vi "MainForceMeasurement.vi"() -> ()   [LabVIEW 2010]
uses:
  <vilib>/Instr/_visa.llb/VISA Flush IO Buffer Mask.ctl
  Variable globale 1.vi
  <vilib>/Instr/_visa.llb/VISA Configure Serial Port (Instr).vi
panel:
  in  "attente (ms)":u32=50
  in  "Temps échelon":i32=25
  out "Sor":string[][](array[string]) caption="Motor torque"
  out "Ent":string[][](array[string]) caption="Motor commande"
  out "Con_XYLeftTorque 2":cluster{"Y":dbl[], "Y":dbl[]}[](graph) caption="Motor Torque"
  out "Con_XYLeftTorque":cluster{"Y":dbl[], "Y":dbl[]}[](graph) caption="Motor  Torque command"
  in  "Temps départ":i32=25
  out "tableau inversé 2":u8[](array[numeric])
  out "tableau inversé":i8[](array[numeric])
  out "error out 2":errorcluster caption="sortie d'erreur"
  in  "Type moteur":i32=139 min=0 max=255
  out "Float recu":sgl
  in  "Couple":sgl=25.45
  out "Iteration 3":i32
  out "Iteration reception":i32
  out "Iteration Envoi":i32
  out "Checksum calculé":i32
  out "Checksum reçu":i32
  out "Type de donnee (ID)":i32
  out "Byte Start ?":bool
  out "Retour 2":string
  in  "stop secu":bool
  in  "STOP":bool
  out "error out":errorcluster caption="sortie d'erreur"
  in  "baud rate (9600)":u32=9600 caption="débit en bauds (9600)"
  in  "Port Com":refnum<visa-resource-name>="COM7" caption="Nom de ressource VISA"
  # "Envoi de l'échelon"
  # "Réception"
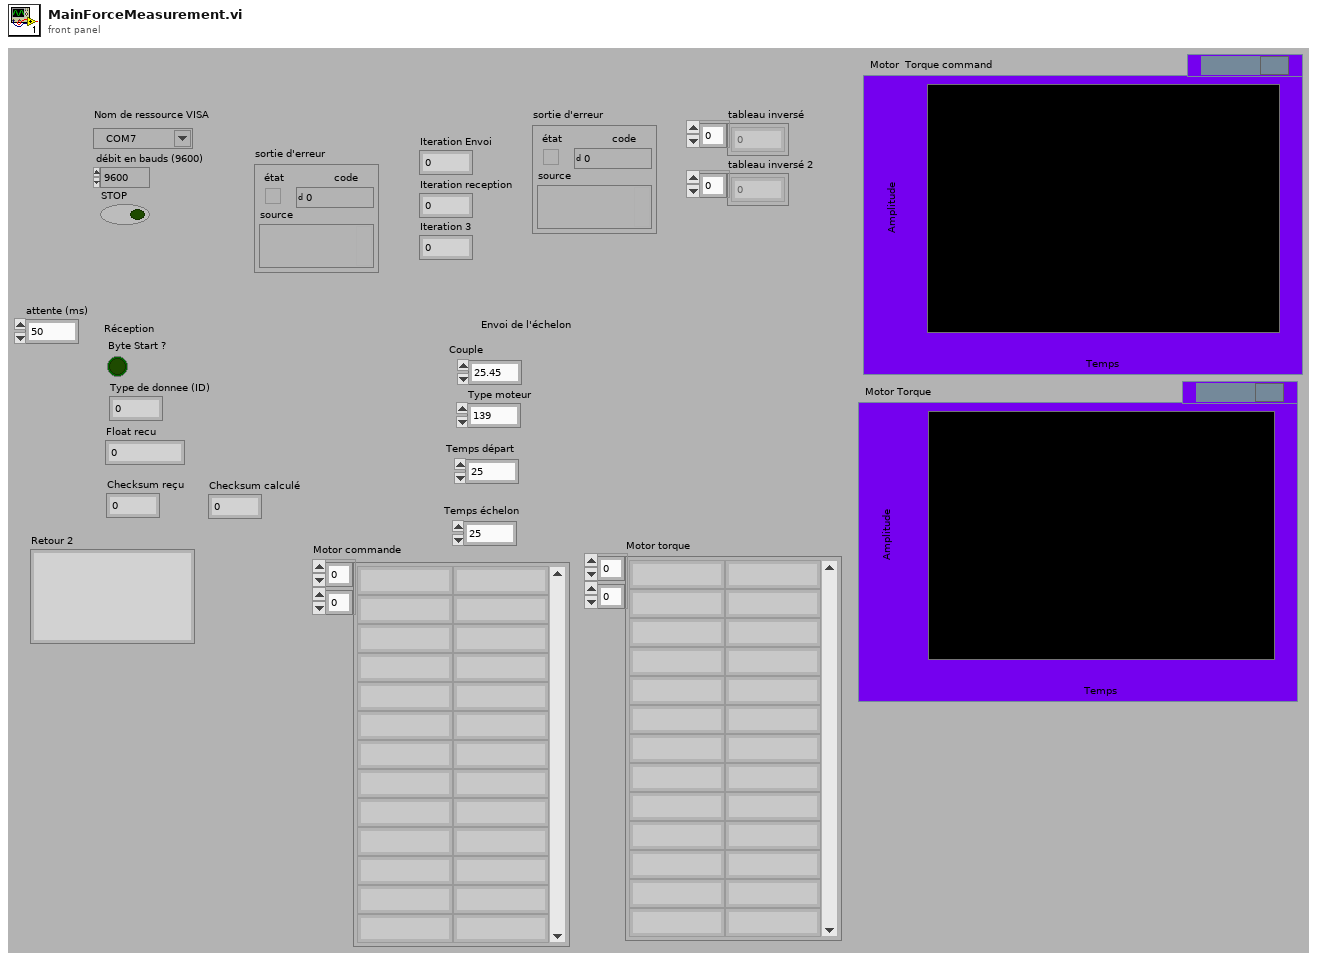
[diagram p1: front panel]
types:
  T1 = typedef "VISA Flush IO Buffer Mask.ctl" = u16
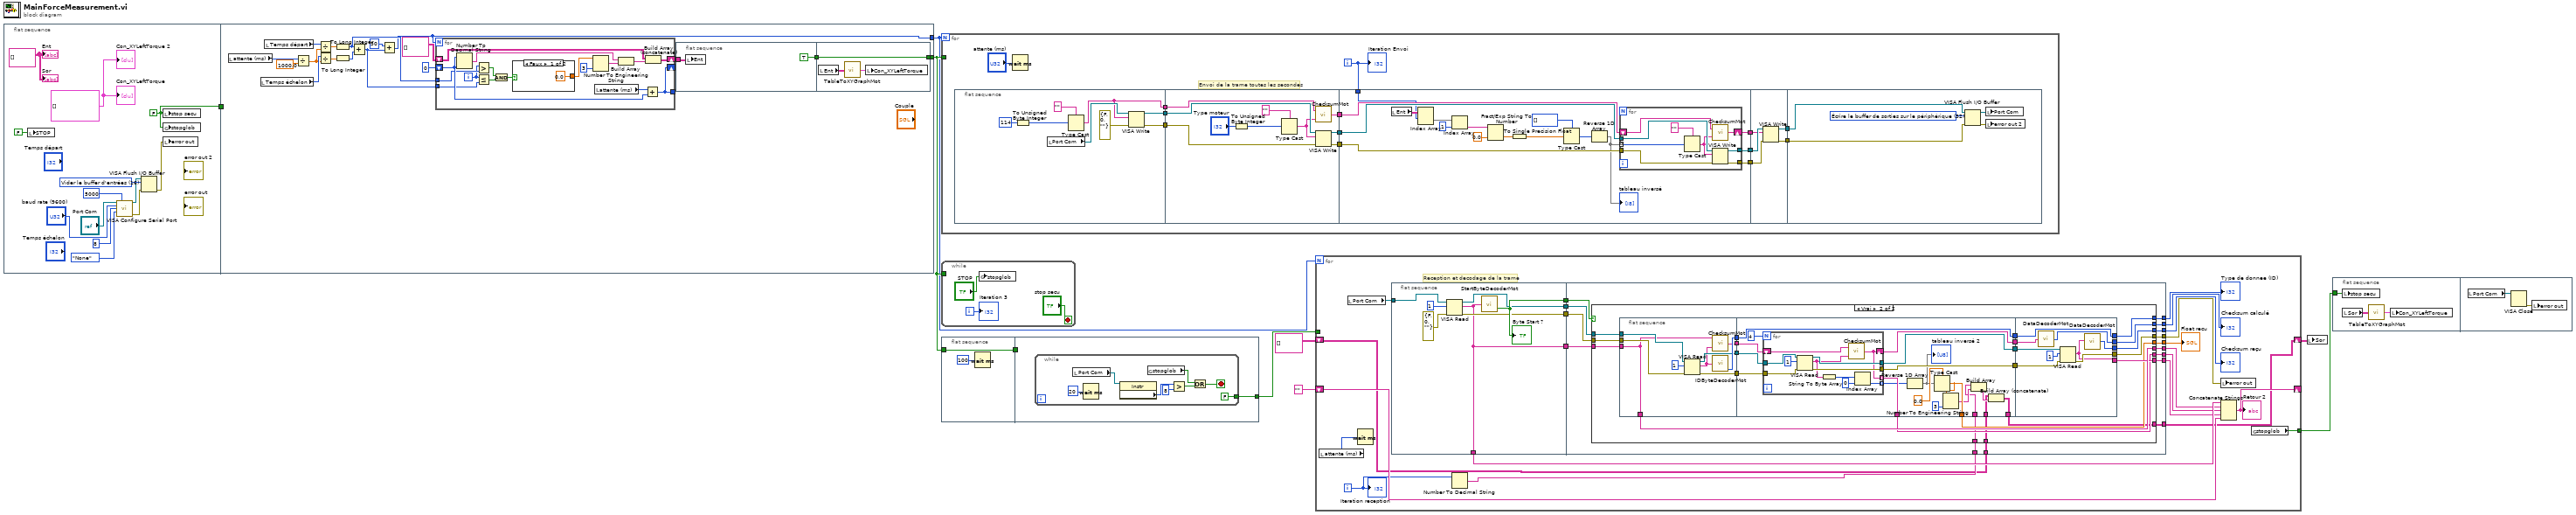
[diagram p0: block diagram]
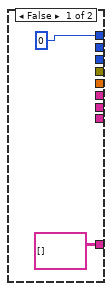
[diagram p2: hidden frame]
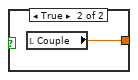
[diagram p3: hidden frame]
diagram:
  n1 = flat-sequence {
    tunnel: [w14] -> w5
    tunnel: [w31] -> w8
    tunnel: w5 -> [_]
    tunnel: [w26] -> w3
    frame #0 {
      w11 = cluster{"Y":dbl[], "Y":dbl[]}[] [] ("Con_XYLeftTorque 2")
      w10 = string[][] [] ("Con_MotorRightTorque")
      w14 = FALSE
      w17 = T1 16 items=["Vider le buffer d'entrées"=16, "Écrire le buffer de sorties sur le périphérique"=32, "Vider le buffer d'entrées (Pas d'E/S)"=64, "Vider le buffer de sorties"=128] ("Mask")
      n2 = local write "STOP"(FALSE) -> ()
      n3 = call-poly "VISA Configure Serial Port"("VISA resource name"="Port Com", "timeout (10sec)"=u32 5000, "baud rate (9600)"="baud rate (9600)", "data bits (8)"=u16 8, "parity (0:none)"=enum16{"None", "Odd", "Even", "Mark", "Space"}."None") -> ("VISA resource name out"=w13:refnum<visa-resource-name>, "error out"=w12:errorcluster)  [unwired: 9 in]
      n4 = VISA Flush I/O Buffer(VISA resource name=w13, mask (16)=w17, error in (no error)=w12) -> (error out=w15:errorcluster)  [unwired: 1 out]
      n5 = local write "stop secu"(w14) -> ()
      n6 = global write "Variable globale 1.vi" "stopglob"(w14) -> ()
      n7 = local write "error out"(w15) -> ()
      "Sor" <- w10
      "Con_XYLeftTorque" <- w11
      "Con_XYLeftTorque 2" <- w11
      "Ent" <- w10
    }
    frame #1 {
      n8 = local read "attente (ms)"() -> (w29:u32)
      n9 = local read "Temps échelon"() -> (w37:i32)
      n10 = local read "Temps départ"() -> (w39:i32)
      n11 = Divide(x=w29, y=sgl 1000.0) -> (x/y=w30:sgl)
      n12 = Divide(x=w39, y=w30) -> (x/y=w38:sgl)
      n13 = Divide(x=w37, y=w30) -> (x/y=w36:sgl)
      n14 = To Long Integer(number=w38) -> (32bit integer=w32:i32)
      n15 = To Long Integer(number=w36) -> (32bit integer=w35:i32)
      n16 = Add(x=w32, y=w35) -> (x+y=w24:i32)
      n17 = Add(x=50, y=w24) -> (x+y=w26:i32)
      n18 = for {
        N: w26 -> [_]
        shift-right: [w51] -> w27
        shift-left: string[][] [] ("Ent") -> [w52]
        shift-right: [w50] -> _
        shift-left: u32 0 -> [w60]
        tunnel: w32 -> [w58]
        tunnel: [w50] -> _
        tunnel: w24 -> [w48]
        i -> [w49]
        n19 = Number To Decimal String(number=w60) -> (decimal integer string=w57:string)  [unwired: 1 in]
        n20 = Greater?(x=w49, y=w58) -> (0:w47:bool)
        n21 = Less Or Equal?(x=w49, y=w48) -> (x <= y?=w46:bool)
        n22 = And(x=w47, y=w46) -> (x .and. y?=w45:bool)
        n23 = case shown="Faux" w45 {
          tunnel: [sgl 0.0 ("Couple") w62] -> w55
          frame False {
          }
          frame True {
            n24 = local read "Couple"() -> (w62:sgl)
          }
        }
        n25 = Number To Engineering String(2:i16 3 ("précision (6)"), 4:w55) -> (0:w56:string)  [unwired: 2 in]
        n26 = local read "attente (ms)"() -> (w59:u32)
        n27 = Build Array(w57, w56) -> (w53:string[])
        n28 = Add(x=w59, y=w60) -> (x+y=w50:u32)
        n29 = Build Array (concatenate)(w52, w53) -> (w51:string[][])
      }
      n30 = flat-sequence {
        tunnel: w27 -> [w40]
        tunnel: [TRUE] -> w23
        tunnel: [w44] -> w31
        tunnel: w23 -> [w44]
        frame #0 {
          n31 = local write "Ent"(w40) -> ()
        }
        frame #1 {
          n32 = local read "Ent"() -> (w42:string[][])
          n33 = call "TableToXYGraphMot.vi"("Input Table"=w42) -> ("XY Graph"=w43:cluster{"Y":dbl[], "Y":dbl[]}[])
          n34 = local write "Con_XYLeftTorque"(w43) -> ()
        }
      }
    }
  }
  n35 = for {
    N: w3 -> [_]
    tunnel: w8 -> [_]
    i -> [w63]
    # "Envoi de la trame toutes les secondes"
    n36 = flat-sequence {
      tunnel: [w80] -> w75
      tunnel: [w79] -> w74
      tunnel: [w78] -> w71
      tunnel: w75 -> [w93]
      tunnel: w74 -> [w92]
      tunnel: [w91] -> w73
      tunnel: [w90] -> w72
      tunnel: w71 -> [w89]
      tunnel: [w88] -> w70
      tunnel: w73 -> [w107]
      tunnel: w72 -> [w109]
      tunnel: w70 -> [w105]
      tunnel: [w108] -> w69
      tunnel: [w106] -> w68
      tunnel: [w104] -> w67
      tunnel: w63 -> [w100]
      tunnel: w69 -> [w124]
      tunnel: w68 -> [w123]
      tunnel: w67 -> [w122]
      tunnel: [w121] -> w65
      tunnel: [w120] -> w64
      tunnel: w65 -> [w129]
      tunnel: w64 -> [w128]
      frame #0 {
        n37 = To Unsigned Byte Integer(number=114) -> (unsigned 8bit integer=w77:u8)
        n38 = local read "Port Com"() -> (w83:refnum<visa-resource-name>)
        n39 = Type Cast(type="", x=w77) -> (*(type *) &x=w78:string)
        n40 = VISA Write(VISA resource name=w83, write buffer=w78, error in (no error)=errorcluster {"status"=FALSE, "code"=0, "source"=""} ("entrée d'erreur (pas d'erreur)")) -> (VISA resource name out=w80:refnum<visa-resource-name>, error out=w79:errorcluster)  [unwired: 1 out]
      }
      frame #1 {
        n41 = To Unsigned Byte Integer(number="Type moteur") -> (unsigned 8bit integer=w86:u8)
        n42 = Type Cast(type="", x=w86) -> (*(type *) &x=w84:string)
        n43 = call "ChecksumMot.vi"("Byte2"=w84, "Byte1"=w89) -> ("chaîne"=w88:string)
        n44 = VISA Write(VISA resource name=w93, write buffer=w84, error in (no error)=w92) -> (VISA resource name out=w90:refnum<visa-resource-name>, error out=w91:errorcluster)  [unwired: 1 out]
      }
      frame #2 {
        n45 = local read "Ent"() -> (w101:string[][])
        n46 = Index Array(array=w101, index (row)=w100) -> (element=w99:string[])  [unwired: 1 in]
        n47 = Index Array(array=w99, index=1 ("indice")) -> (element=w97:string)
        n48 = Fract/Exp String To Number(string=w97, default (0 dbl)=0.0 ("valeur par défaut (0 DBL)")) -> (number=w95:dbl)  [unwired: 2 in, 1 out]
        n49 = To Single Precision Float(number=w95) -> (single precision float=w94:sgl)
        n50 = Type Cast(type=i8[] [] ("tableau d'octets non signés"), x=w94) -> (*(type *) &x=w103:i8[])
        n51 = Reverse 1D Array(array=w103) -> (reversed array=w102:i8[])
        "tableau inversé" <- w102
        n52 = for {
          tunnel: w102 -> [w119] mode=indexing
          tunnel: w109 -> [w117]
          tunnel: [w116] -> w108
          tunnel: w107 -> [w115]
          tunnel: [w114] -> w106
          shift-right: [w111] -> w104
          shift-left: w105 -> [w113]
          n53 = Type Cast(type="", x=w119) -> (*(type *) &x=w112:string)
          n54 = call "ChecksumMot.vi"("Byte2"=w112, "Byte1"=w113) -> ("chaîne"=w111:string)
          n55 = VISA Write(VISA resource name=w117, write buffer=w112, error in (no error)=w115) -> (VISA resource name out=w116:refnum<visa-resource-name>, error out=w114:errorcluster)  [unwired: 1 out]
        }
      }
      frame #3 {
        n56 = VISA Write(VISA resource name=w124, write buffer=w122, error in (no error)=w123) -> (VISA resource name out=w121:refnum<visa-resource-name>, error out=w120:errorcluster)  [unwired: 1 out]
      }
      frame #4 {
        w125 = T1 32 items=["Vider le buffer d'entrées"=16, "Écrire le buffer de sorties sur le périphérique"=32, "Vider le buffer d'entrées (Pas d'E/S)"=64, "Vider le buffer de sorties"=128] ("Mask")
        n57 = VISA Flush I/O Buffer(VISA resource name=w129, mask (16)=w125, error in (no error)=w128) -> (VISA resource name out=w126:refnum<visa-resource-name>, error out=w127:errorcluster)
        n58 = local write "Port Com"(w126) -> ()
        n59 = local write "error out 2"(w127) -> ()
      }
    }
    n60 = Wait (ms)(milliseconds to wait="attente (ms)") -> ()  [unwired: 1 out]
    "Iteration Envoi" <- w63
  }
  n61 = while {
    tunnel: w8 -> [_]
    i -> [w130]
    stop <- "stop secu" stop-if-true
    n62 = global write "Variable globale 1.vi" "stopglob"("STOP") -> ()
    "Iteration 3" <- w130
  }
  n63 = flat-sequence {
    tunnel: w8 -> [w133]
    tunnel: [w133] -> w7
    tunnel: w7 -> [_]
    tunnel: [w135] -> w6
    frame #0 {
      n64 = Wait (ms)(milliseconds to wait=u32 100 ("attente (ms)")) -> ()  [unwired: 1 out]
    }
    frame #1 {
      n65 = while {
        tunnel: [FALSE] -> w135
        stop <- w142 stop-if-true
        n66 = local read "Port Com"() -> (w141:refnum<visa-resource-name>)
        n67 = Wait (ms)(milliseconds to wait=u32 20 ("attente (ms)")) -> ()  [unwired: 1 out]
        n68 = property class="Instr"(reference=w141) -> ("Serial Settings:Number of Bytes at Serial Port"=w140:u32)  [unwired: 1 in, 2 out]
        n69 = global read "Variable globale 1.vi" "stopglob"() -> (w143:bool)
        n70 = Greater?(x=w140, y=u32 8) -> (0:w138:bool)
        n71 = Or(x=w143, y=w138) -> (x .or. y?=w142:bool)
      }
    }
  }
  n72 = for {
    N: w3 -> [_]
    shift-right: [w151] -> _
    shift-left: "" -> [w152]
    tunnel: w6 -> [_]
    tunnel: [w148] -> w4
    shift-right: [w144] -> w1
    shift-left: string[][] [] ("Sor") -> [w145]
    i -> [w147]
    # "Reception et decodage de la trame"
    n73 = local read "attente (ms)"() -> (w165:u32)
    n74 = local read "Port Com"() -> (w164:refnum<visa-resource-name>)
    n75 = Wait (ms)(milliseconds to wait=w165) -> ()  [unwired: 1 out]
    n76 = flat-sequence {
      tunnel: w164 -> [w171]
      tunnel: [w170] -> w163
      tunnel: [w169] -> w162
      tunnel: [w168] -> w161
      tunnel: [w167] -> w159
      tunnel: [w167] -> w155
      tunnel: w163 -> [w187]
      tunnel: w162 -> [w186]
      tunnel: w161 -> [w185]
      tunnel: [w184] -> w160
      tunnel: w159 -> [w183]
      tunnel: [w182] -> w158
      tunnel: [w181] -> w157
      tunnel: [w180] -> w156
      tunnel: [w179] -> w154
      tunnel: [w178] -> w153
      tunnel: [w177] -> w150
      tunnel: [w176] -> w149
      tunnel: w146 -> [w175]
      tunnel: w145 -> [w174]
      tunnel: [w173] -> w144
      frame #0 {
        n77 = VISA Read(VISA resource name=w171, byte count=u32 1 ("nombre d'octets"), error in (no error)=errorcluster {"status"=FALSE, "code"=0, "source"=""} ("entrée d'erreur (pas d'erreur)")) -> (VISA resource name out=w169:refnum<visa-resource-name>, read buffer=w167:string, error out=w168:errorcluster)  [unwired: 1 out]
        n78 = call "StartByteDecoderMot.vi"("byte1"=w167) -> ("Byte Start ?"=w170:bool)  [unwired: 1 in]
        "Byte Start ?" <- w170
      }
      frame #1 {
        n79 = case shown="Vrai" w187 {
          tunnel: w186 -> [_ w211]
          tunnel: w185 -> [_ w210]
          tunnel: [0 ("Type de donnee (ID)") w209] -> w184
          tunnel: w183 -> [_ w204]
          tunnel: [_ w202] -> w182
          tunnel: [_ w201] -> w181
          tunnel: [_ w200] -> w180
          tunnel: [_ w199] -> w179
          tunnel: [_ w198] -> w178
          tunnel: [_ w195] -> w177
          tunnel: [_ w193] -> w176
          tunnel: w175 -> [_ w192]
          tunnel: w174 -> [_ w191]
          tunnel: [string[][] [] w190] -> w173
          frame False {
          }
          frame True {
            n80 = flat-sequence {
              tunnel: w211 -> [w220]
              tunnel: w210 -> [w219]
              tunnel: [w217] -> w208
              tunnel: [w216] -> w207
              tunnel: [w215] -> w206
              tunnel: w204 -> [w212]
              tunnel: [w213] -> w203
              tunnel: [w212] -> w199
              tunnel: w208 -> [w239]
              tunnel: w207 -> [w238]
              tunnel: w206 -> [w235]
              tunnel: [w239] -> w205
              tunnel: w203 -> [w233]
              tunnel: [w237] -> w197
              tunnel: [w236] -> w196
              tunnel: [w227] -> w195
              tunnel: [w232] -> w194
              tunnel: [w230] -> w193
              tunnel: w192 -> [w224]
              tunnel: w191 -> [w222]
              tunnel: [w221] -> w190
              tunnel: [w259] -> w209
              tunnel: w205 -> [w259]
              tunnel: [w257] -> w202
              tunnel: [w256] -> w201
              tunnel: [w255] -> w200
              tunnel: [w254] -> w198
              tunnel: w197 -> [w253]
              tunnel: w196 -> [w252]
              tunnel: w194 -> [w251]
              frame #0 {
                n81 = VISA Read(VISA resource name=w220, byte count=u32 1 ("nombre d'octets"), error in (no error)=w219) -> (VISA resource name out=w216:refnum<visa-resource-name>, read buffer=w214:string, error out=w215:errorcluster)  [unwired: 1 out]
                n82 = call "ChecksumMot.vi"("Byte2"=w214, "Byte1"=w212) -> ("chaîne"=w213:string)
                n83 = call "IDByteDecoderMot.vi"("byte1"=w214) -> ("Type de donnee (ID)"=w217:i32)  [unwired: 2 out]
              }
              frame #1 {
                n84 = for {
                  N: 4 -> [_]
                  tunnel: w238 -> [w249]
                  tunnel: [w248] -> w237
                  tunnel: [w247] -> w236
                  tunnel: w235 -> [w246]
                  tunnel: [w243] -> w229 mode=indexing
                  shift-right: [w240] -> w232
                  shift-left: w233 -> [w242]
                  tunnel: [w240] -> w230 mode=indexing
                  n85 = VISA Read(VISA resource name=w249, byte count=u32 1 ("nombre d'octets"), error in (no error)=w246) -> (VISA resource name out=w248:refnum<visa-resource-name>, read buffer=w241:string, error out=w247:errorcluster)  [unwired: 1 out]
                  n86 = String To Byte Array(string=w241) -> (unsigned byte array=w245:u8[])
                  n87 = call "ChecksumMot.vi"("Byte2"=w241, "Byte1"=w242) -> ("chaîne"=w240:string)
                  n88 = Index Array(array=w245, index=0 ("indice")) -> (element=w243:u8)
                }
                n89 = Reverse 1D Array(array=w229) -> (reversed array=w228:u8[])
                "tableau inversé 2" <- w228
                n90 = Type Cast(type=sgl 0.0, x=w228) -> (*(type *) &x=w227:sgl)
                n91 = Number To Engineering String(2:i16 3 ("précision (6)"), 4:w227) -> (0:w225:string)  [unwired: 2 in]
                n92 = Build Array(w224, w225) -> (w223:string[])
                n93 = Build Array (concatenate)(w222, w223) -> (w221:string[][])
              }
              frame #2 {
                n94 = call "DataDecoderMot.vi"("byte1"=w251) -> ("Data"=w257:i32)
                n95 = VISA Read(VISA resource name=w253, byte count=u32 1 ("nombre d'octets"), error in (no error)=w252) -> (read buffer=w254:string, error out=w255:errorcluster)  [unwired: 2 out]
                n96 = call "DataDecoderMot.vi"("byte1"=w254) -> ("Data"=w256:i32)
              }
            }
          }
        }
      }
    }
    n97 = Number To Decimal String(number=w147) -> (decimal integer string=w146:string)  [unwired: 1 in]
    n98 = local write "error out"(w156) -> ()
    n99 = Concatenate Strings(w155, w154, w149, w153, w152) -> (w151:string)
    "Retour 2" <- w151
    n100 = global read "Variable globale 1.vi" "stopglob"() -> (w148:bool)
    "Type de donnee (ID)" <- w160
    "Checksum reçu" <- w157
    "Checksum calculé" <- w158
    "Iteration reception" <- w147
    "Float recu" <- w150
  }
  n101 = local write "Sor"(w1) -> ()
  n102 = flat-sequence {
    tunnel: w4 -> [w262]
    frame #0 {
      n103 = local write "stop secu"(w262) -> ()
      n104 = local read "Sor"() -> (w261:string[][])
      n105 = call "TableToXYGraphMot.vi"("Input Table"=w261) -> ("XY Graph"=w260:cluster{"Y":dbl[], "Y":dbl[]}[])
      n106 = local write "Con_XYLeftTorque"(w260) -> ()
    }
    frame #1 {
      n107 = local read "Port Com"() -> (w264:refnum<visa-resource-name>)
      n108 = VISA Close(VISA resource name=w264) -> (error out=w263:errorcluster)  [unwired: 1 in]
      n109 = local write "error out"(w263) -> ()
    }
  }
